vi "resetOutput.vi"(8 "error in (no error)":errorcluster, 11 "niDAQmxAO in":refnum<class "niDAQmxAO.lvclass">) -> (0 "error out":errorcluster, 3 "niDAQmxAO out":refnum<class "niDAQmxAO.lvclass">)   [LabVIEW 2009, in "Hardware.lvlib" / "Channels.lvlib" / "niDAQmxAO.lvclass"]
uses:
  niDAQmxAO.lvclass
  <vilib>/DAQmx/write.llb/DAQmx Write (Analog 1D DBL NChan 1Samp).vi
  <vilib>/DAQmx/create/channels.llb/DAQmx Create Channel (AO-Voltage-Basic).vi
  AnalogOutput.lvclass
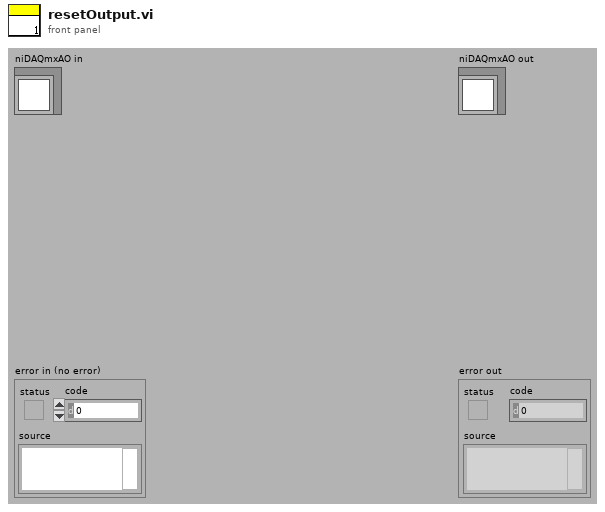
[diagram p1: front panel]
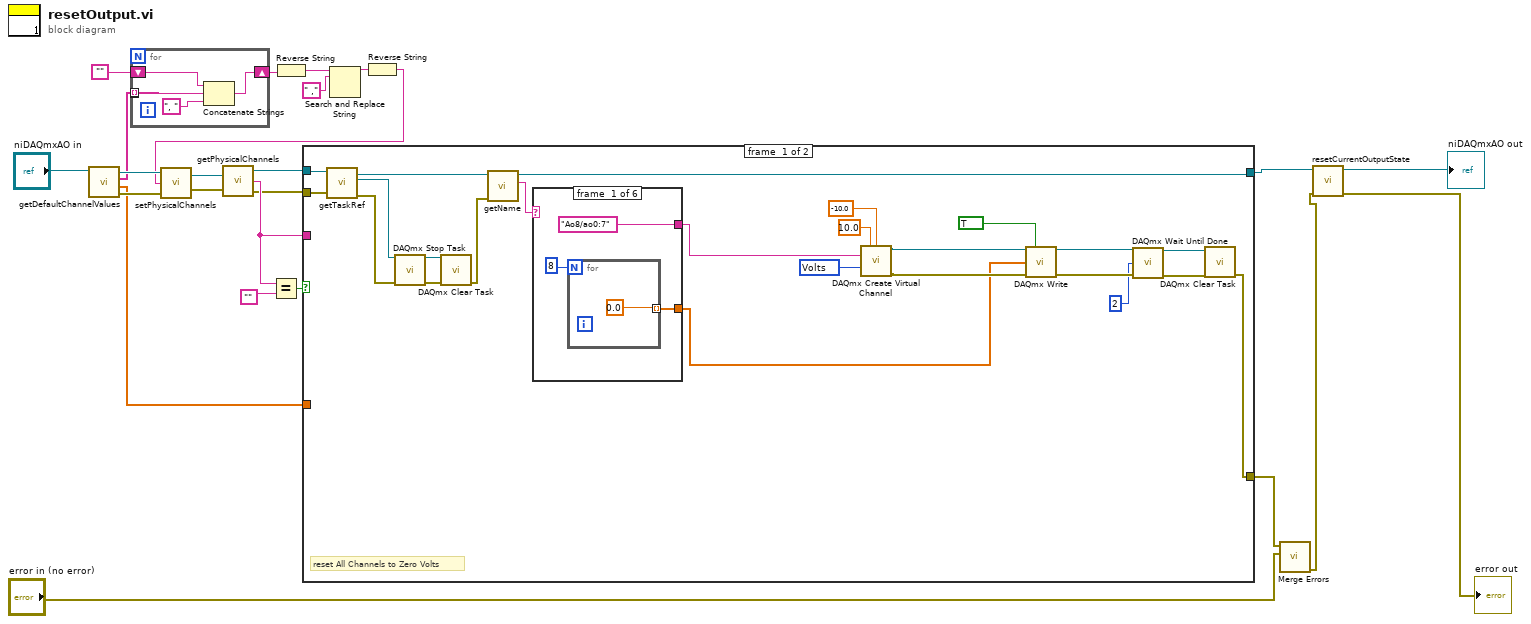
[diagram p0: block diagram]
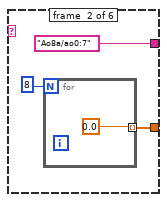
[diagram p2: hidden frame]
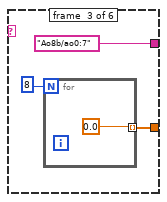
[diagram p3: hidden frame]
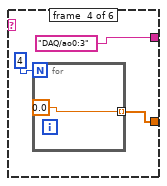
[diagram p4: hidden frame]
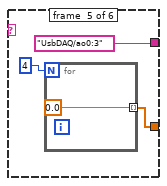
[diagram p5: hidden frame]
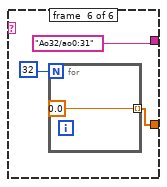
[diagram p6: hidden frame]
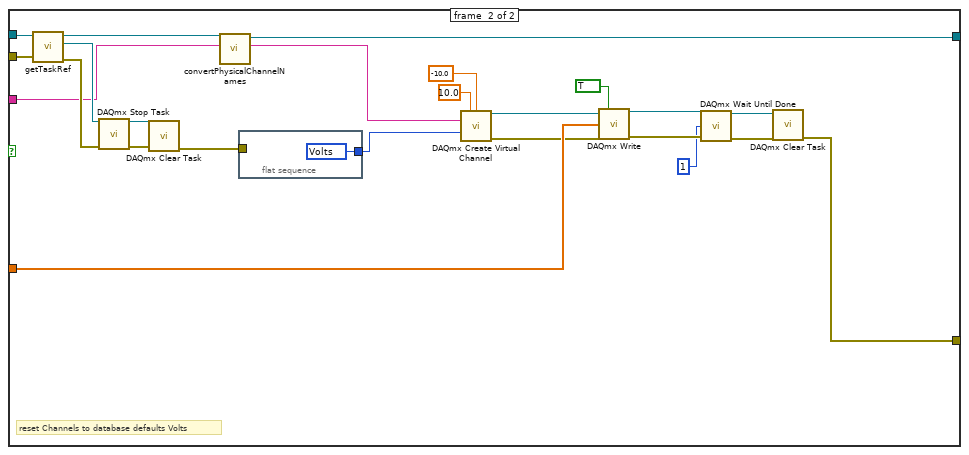
[diagram p7: hidden frame]
diagram:
  n1 = call "getDefaultChannelValues.vi"("AnalogOutput in"="niDAQmxAO in") -> ("error out"=w6:errorcluster, "calibratedValues"=w5:dbl[], "channel_addresses"=w13:string[], "AnalogOutput out"=w16:refnum<class "niDAQmxAO.lvclass">)  [unwired: 7 in]
  n2 = for {
    tunnel: [w27] -> _ mode=indexing
    tunnel: w13 -> [w27] mode=indexing
    shift-right: [w25] -> w11
    shift-left: "" -> [w28]
    n3 = Concatenate Strings(w28, w27, ", ") -> (w25:string)
  }
  n4 = Reverse String(1:w11) -> (0:w10:string)
  n5 = Search and Replace String(input string=w10, search string=" ,") -> (result string=w8:string)  [unwired: 6 in, 3 out]
  n6 = Reverse String(1:w8) -> (0:w7:string)
  n7 = call-dynamic "setPhysicalChannels.vi"("error in (no error)"=w6, "Physical Channels"=w7, "AnalogOutput.lvclass in"=w16) -> ("error out"=w14:errorcluster, "AnalogOutput.lvclass out"=w15:refnum<class "niDAQmxAO.lvclass">)
  n8 = call-dynamic "getPhysicalChannels.vi"("AnalogOutput.lvclass in"=w15, "error in (no error)"=w14) -> ("AnalogOutput.lvclass out"=w21:refnum<class "niDAQmxAO.lvclass">, "Physical Channels"=w22:string, "error out"=w20:errorcluster)
  n9 = Equal?(x=w22, y="") -> (x = y?=w23:bool)
  n10 = case shown="False" w23 {
    tunnel: w22 -> [_ w83]
    tunnel: w21 -> [w52 w100]
    tunnel: [w44 w81] -> w4
    tunnel: w20 -> [w51 w99]
    tunnel: [w37 w89] -> w19
    tunnel: w5 -> [_ w79]
    frame #0 {
      w29 = 10348 items=["Volts"=10348, "From Custom Scale"=10065] ("units")
      # "reset All Channels to Zero Volts"
      n11 = call "getTaskRef.vi"("error in (no error)"=w51, "niDAQmxAO.lvclass in"=w52) -> ("error out"=w49:errorcluster, "DAQmx Task Ref"=w50:refnum<k21>, "niDAQmxAO.lvclass out"=w46:refnum<class "niDAQmxAO.lvclass">)  [unwired: 7 in]
      n12 = call <vilib>:"DAQmx Stop Task.vi"("task/channels in"=w50, "error in"=w49) -> ("task out"=w48:refnum<k21>, "error out"=w47:errorcluster)  [unwired: 12 in]
      n13 = call <vilib>:"DAQmx Clear Task.vi"("task in"=w48, "error in"=w47) -> ("error out"=w45:errorcluster)  [unwired: 13 in]
      n14 = call "getName.vi"("error in (no error)"=w45, "AnalogOutput.lvclass in"=w46) -> ("name"=w43:string, "AnalogOutput.lvclass out"=w44:refnum<class "niDAQmxAO.lvclass">)  [unwired: 7 in, 1 out]
      n15 = case shown="\"Ao8a\"" w43 {
        tunnel: ["Ao8/ao0:7" "Ao8a/ao0:7" "Ao8b/ao0:7" "DAQ/ao0:3" "UsbDAQ/ao0:3" "Ao32/ao0:31"] -> w30
        tunnel: [w53 w57 w61 w65 w69 w73] -> w31
        frame #0 {
          n16 = for {
            N: 8 -> [_]
            tunnel: [0.0] -> w53 mode=indexing
          }
        }
        frame #1 {
          n17 = for {
            N: 8 -> [_]
            tunnel: [0.0] -> w57 mode=indexing
          }
        }
        frame #2 {
          n18 = for {
            N: 8 -> [_]
            tunnel: [0.0] -> w61 mode=indexing
          }
        }
        frame #3 {
          n19 = for {
            N: 4 -> [_]
            tunnel: [0.0] -> w65 mode=indexing
          }
        }
        frame #4 {
          n20 = for {
            N: 4 -> [_]
            tunnel: [0.0] -> w69 mode=indexing
          }
        }
        frame #5 {
          n21 = for {
            N: 32 -> [_]
            tunnel: [0.0] -> w73 mode=indexing
          }
        }
      }
      n22 = call-poly <vilib>:"DAQmx Create Virtual Channel.vi"("maximum value"=10.0, "minimum value"=-10.0, "physical channels"=w30, "units"=w29) -> ("task out"=w33:refnum<k21>, "error out"=w32:errorcluster)  [unwired: 10 in]
      n23 = call-poly <vilib>:"DAQmx Write.vi"("task/channels in"=w33, "auto start"=TRUE, "data"=w31, "error in"=w32) -> ("task out"=w41:refnum<k21>, "error out"=w40:errorcluster)  [unwired: 9 in, 1 out]
      n24 = call <vilib>:"DAQmx Wait Until Done.vi"("task/channels in"=w41, "timeout (sec)"=2, "error in"=w40) -> ("task out"=w39:refnum<k21>, "error out"=w38:errorcluster)  [unwired: 11 in]
      n25 = call <vilib>:"DAQmx Clear Task.vi"("task in"=w39, "error in"=w38) -> ("error out"=w37:errorcluster)  [unwired: 13 in]
    }
    frame #1 {
      # "reset Channels to database defaults Volts"
      n26 = call "getTaskRef.vi"("error in (no error)"=w99, "niDAQmxAO.lvclass in"=w100) -> ("error out"=w97:errorcluster, "DAQmx Task Ref"=w98:refnum<k21>, "niDAQmxAO.lvclass out"=w82:refnum<class "niDAQmxAO.lvclass">)  [unwired: 7 in]
      n27 = call <vilib>:"DAQmx Stop Task.vi"("task/channels in"=w98, "error in"=w97) -> ("task out"=w88:refnum<k21>, "error out"=w87:errorcluster)  [unwired: 12 in]
      n28 = call <vilib>:"DAQmx Clear Task.vi"("task in"=w88, "error in"=w87) -> ("error out"=w86:errorcluster)  [unwired: 13 in]
      n29 = call "convertPhysicalChannelNames.vi"("PhysicalChannels"=w83, "niDAQmxAO.lvclass in"=w82) -> ("channel_names"=w80:string, "niDAQmxAO.lvclass out"=w81:refnum<class "niDAQmxAO.lvclass">)  [unwired: 7 in, 1 out]
      n30 = flat-sequence {
        tunnel: w86 -> [_]
        tunnel: [w101] -> w85
        frame #0 {
          w101 = 10348 items=["Volts"=10348, "From Custom Scale"=10065] ("units")
        }
      }
      n31 = call-poly <vilib>:"DAQmx Create Virtual Channel.vi"("maximum value"=10.0, "minimum value"=-10.0, "physical channels"=w80, "units"=w85) -> ("task out"=w78:refnum<k21>, "error out"=w77:errorcluster)  [unwired: 10 in]
      n32 = call-poly <vilib>:"DAQmx Write.vi"("task/channels in"=w78, "auto start"=TRUE, "data"=w79, "error in"=w77) -> ("task out"=w93:refnum<k21>, "error out"=w92:errorcluster)  [unwired: 9 in, 1 out]
      n33 = call <vilib>:"DAQmx Wait Until Done.vi"("task/channels in"=w93, "timeout (sec)"=1, "error in"=w92) -> ("task out"=w91:refnum<k21>, "error out"=w90:errorcluster)  [unwired: 11 in]
      n34 = call <vilib>:"DAQmx Clear Task.vi"("task in"=w91, "error in"=w90) -> ("error out"=w89:errorcluster)  [unwired: 13 in]
    }
  }
  n35 = call <vilib>:"Merge Errors.vi"("error in 2 (no error)"="error in (no error)", "error in 1 (no error)"=w19) -> ("error out"=w2:errorcluster)  [unwired: 5 in]
  n36 = call "resetCurrentOutputState.vi"("error in (no error)"=w2, "AnalogOutput in"=w4) -> ("error out"=→"error out":errorcluster, "AnalogOutput out"=→"niDAQmxAO out":refnum<class "niDAQmxAO.lvclass">)  [unwired: 8 in]
